vi "AddEntry.vi"(7 "Index":i32, 8 "error in (no error)":errorcluster, 9 "name":string, 10 "Game in":refnum<class "Game.lvclass">, 11 "Highscore in":refnum<class "Highscore.lvclass">) -> (0 "error out":errorcluster, 2 "Game out":refnum<class "Game.lvclass">, 3 "Highscore out":refnum<class "Highscore.lvclass">)   [LabVIEW 2019, in "RT_Game.lvlib" / "Highscore.lvclass"]
uses:
  Highscore.lvclass
  Game/Game.lvclass
  Highscore.lvclass/Highscore.ctl
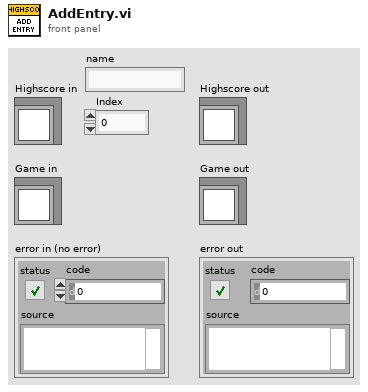
[diagram p1: front panel]
types:
  T1 = typedef "RT_Game.lvlib/Highscore.lvclass/HighscoreEntry.ctl" = cluster{"Name":string, "Score":dbl}
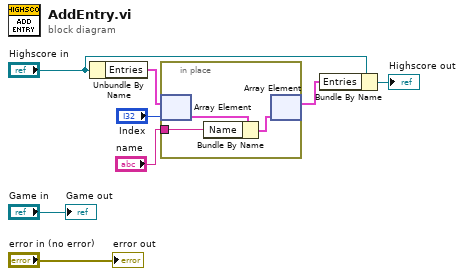
[diagram p0: block diagram]
diagram:
  n1 = Unbundle By Name("Highscore in") -> ("Entries"=w5:T1[])
  n2 = in-place {
    in-place-border: "name" -> [w9]
    n3 = in-place-array #1(w5, "Index") -> (w11:T1)
    n4 = Bundle By Name(cluster=w11, "Name"=w9) -> (w10:T1)
    n5 = in-place-array #1(w10) -> (w3:T1[])  [unwired: 1 out]
  }
  n6 = Bundle By Name(cluster="Highscore in", "Entries"=w3) -> (→"Highscore out":refnum<class "Highscore.lvclass">)
  "Game out" <- "Game in"
  "error out" <- "error in (no error)"
